vi "G# - DependencyInjectionUsingDefaultConstructor.vi"() -> ()   [LabVIEW 2020]
doc: "Dependency Injection wiith G# Default Constructor\nThis examples demonstrates how the default constructor works. This type of implementation can be used to create a injection/plug in pattern when building architectures.\n\nBy using the G# Debugger found in Tools->G# Debugger a text log can be followed showing how the objects were created and destroyed."
uses:
  MyG#SubClass_class/MyG#SubClass.lvclass
  MyG#Class_class/MyG#Class.lvclass
  <vilib>/addons/_AddQ/G#Object/G#Object.lvclass
panel:
  in  "error in":errorcluster
  in  "MySubAttribute in":dbl=5.0
  in  "My Attribute in":dbl=2.0
  out "MyAttribute":dbl
  out "class name":string
  out "class path":path
  out "error out":errorcluster
  out "OK":bool
  out "# of objects killed":i32
  # "Dependency Injection with G# Default Constructor\nThis examples demonstrates how the default constructor works. This type of implementation can be used to create a injection/plug-in\npattern when building architectures.\n\nBy using the G# Debugger found in Tools->G# Debugger a text log can be followed showing how the objects were created and destroyed."
  # "Constructor parameters"
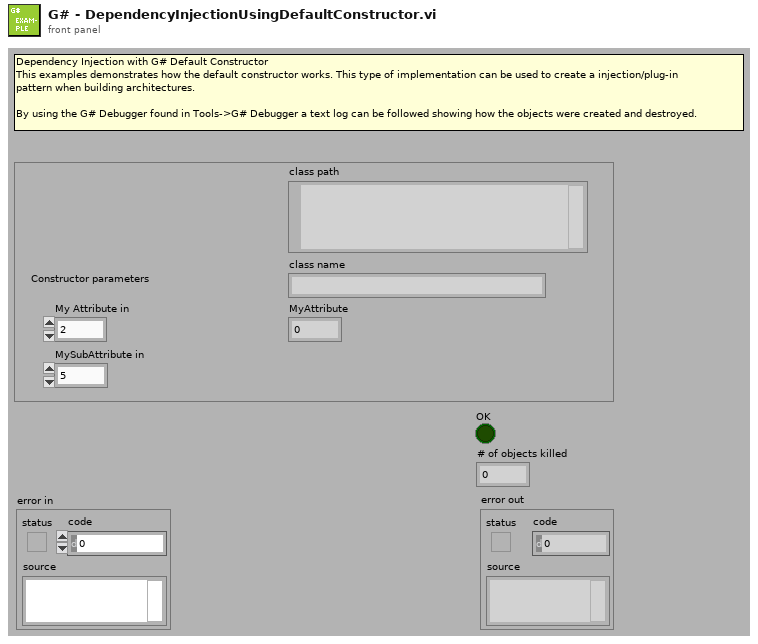
[diagram p1: front panel]
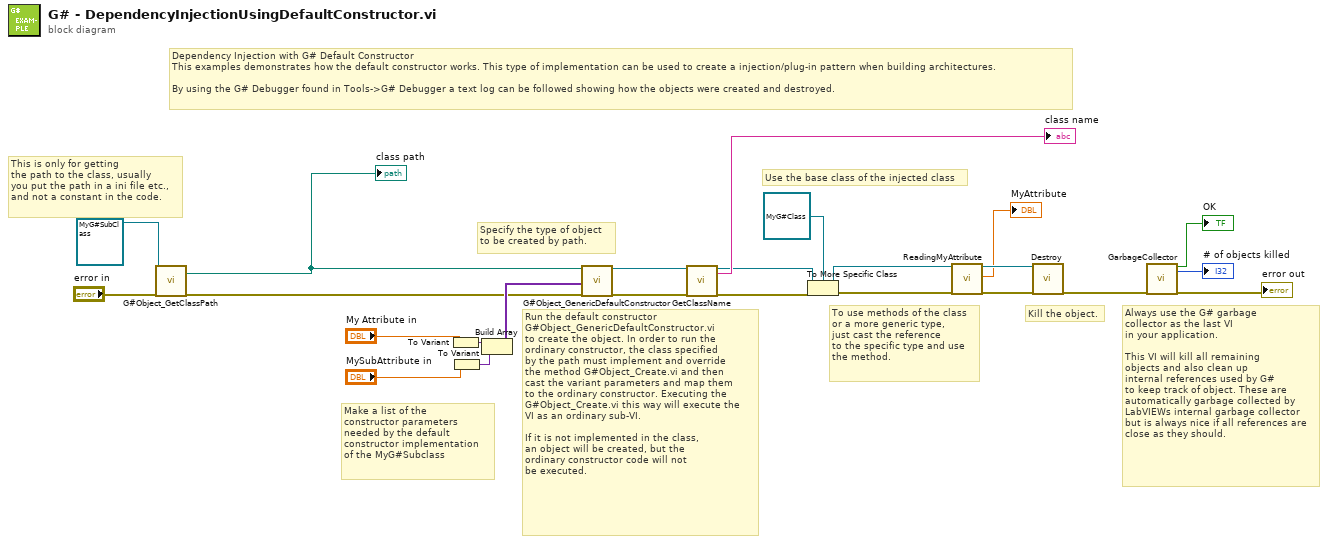
[diagram p0: block diagram]
diagram:
  # "Use the base class of the injected class"
  # "Specify the type of object\nto be created by path."
  # "This is only for getting\nthe path to the class, usually\nyou put the path in a ini file etc.,\nand not a constant in the code."
  # "Dependency Injection with G# Default Constructor\nThis examples demonstrates how the default constructor works. This type of implementation can be used to create a injection/plug-in pattern when building architectures.\n\nBy using the G# Debugger found in Tools->G# Debugger a text log can be followed showing how the objects were created and destroyed."
  # "To use methods of the class\nor a more generic type,\njust cast the reference\nto the specific type and use\nthe method."
  # "Kill the object."
  # "Make a list of the \nconstructor parameters\nneeded by the default\nconstructor implementation\nof the MyG#Subclass"
  # "Run the default constructor\nG#Object_GenericDefaultConstructor.vi\nto create the object. In order to run the\nordinary constructor, the class specified\nby the path must implement and override\nthe method G#Object_Create.vi and then\ncast the variant parameters and map them\nto the ordinary constructor. Executing the\nG#Object_Create.vi this way will execute the\nVI as an ordinary sub-VI.\n\nIf it is not implemented in the class,\nan object will be created, but the\nordinary constructor code will not\nbe executed."
  # "Always use the G# garbage\ncollector as the last VI\nin your application.\n\nThis VI will kill all remaining\nobjects and also clean up\ninternal references used by G#\nto keep track of object. These are\nautomatically garbage collected by\nLabVIEWs internal garbage collector\nbut is always nice if all references are\nclose as they should."
  n1 = call-dynamic "G#Object_GetClassPath.vi"("reference in"=refnum<class "MyG#SubClass.lvclass"> refnum ("MyG#SubClass.lvclass"), "error in (no error)"="error in") -> ("class path"=w9:path, "error out"=w10:errorcluster)  [unwired: 15 in, 1 out]
  "class path" <- w9
  n2 = To Variant(anything="My Attribute in") -> (Variant=w18:variant)
  n3 = To Variant(anything="MySubAttribute in") -> (Variant=w17:variant)
  n4 = Build Array(w18, w17) -> (w14:variant[])
  n5 = call <vilib>:"G#Object_GenericDefaultConstructor.vi"("class path"=w9, "control values"=w14, "error in (no error)"=w10) -> ("reference out"=w2:refnum<class "G#Object.lvclass">, "error out"=w1:errorcluster)  [unwired: 14 in, 1 out]
  n6 = call-dynamic "GetClassName.vi"("reference in"=w2, "error in (no error)"=w1) -> ("reference out"=w11:refnum<class "G#Object.lvclass">, "class name"=→"class name":string, "error out"=w13:errorcluster)  [unwired: 13 in, 2 out]
  n7 = To More Specific Class(target class=refnum<class "MyG#Class.lvclass"> refnum ("MyG#Class.lvclass"), reference=w11, error in=w13) -> (specific class reference=w3:refnum<class "MyG#Class.lvclass">, error out=w4:errorcluster)
  n8 = call-dynamic "ReadingMyAttribute.vi"("reference in"=w3, "error in (no error)"=w4) -> ("reference out"=w6:refnum<class "MyG#Class.lvclass">, "MyAttribute"=→"MyAttribute":dbl, "error out"=w7:errorcluster)  [unwired: 15 in]
  n9 = call-dynamic "Destroy.vi"("reference in"=w6, "error in (no error)"=w7) -> ("error out"=w22:errorcluster)  [unwired: 16 in, 1 out]
  n10 = call <vilib>:"GarbageCollector.vi"("error in (no error)"=w22) -> ("OK"=→"OK":bool, "# of objects killed"=→"# of objects killed":i32, "error out"=→"error out":errorcluster)  [unwired: 16 in]
